vi "get settings directory.vi"() -> (0 "settings directory":path)   [LabVIEW 2014, in "PTUtils.lvlib"]
uses:
  PTUtils.lvlib
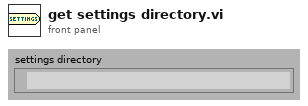
[diagram p1: front panel]
types:
  T1 = enum32{"invalid app kind", "Development System", "Run Time System", "Student Edition", "Embedded LabVIEW", "Evaluation", "Custom"}
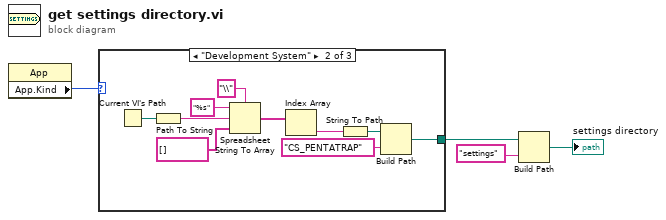
[diagram p0: block diagram]
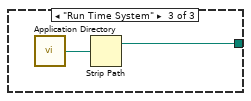
[diagram p3: hidden frame]
diagram:
  n1 = property class="App"() -> ("App.Kind"=w4:T1)  [unwired: 2 in, 2 out]
  n2 = case shown="\"Development System\"" w4 {
    tunnel: [_ w5 w15] -> w2
    frame "invalid app kind", Default {
    }
    frame "Development System" {
      n3 = Current VI's Path() -> (path=w14:path)
      n4 = Path To String(path=w14) -> (string=w13:string)
      n5 = Spreadsheet String To Array(delimiter (Tab)="\\", format string="%s", spreadsheet string=w13, array type (2D Dbl)=string[] []) -> (array=w9:string[])
      n6 = Index Array(array=w9) -> (element=w8:string)  [unwired: 1 in]
      n7 = String To Path(string=w8) -> (path=w7:path)
      n8 = Build Path(base path=w7, name or relative path="CS_PENTATRAP") -> (appended path=w5:path)
    }
    frame "Run Time System" {
      n9 = call <vilib>:"Application Directory.vi"() -> ("Application Directory"=w16:path)
      n10 = Strip Path(path=w16) -> (stripped path=w15:path)  [unwired: 1 out]
    }
  }
  n11 = Build Path(base path=w2, name or relative path="settings") -> (appended path=→"settings directory":path)
